vi "SplashWindow.vi"(7 "Name (\"\" to Use UUID)":string="SplashWindow") -> ()   [LabVIEW 2020, in "CSM-SplashWindow.lvlib"]
doc: "------------- lvcsm -------------\n[CSMStates]\nItem 0 = \"Idle\"\nItem 1 = \"CSM Documentation\"\nItem 2 = \"VI Reference\"\nItem 3 = \"Error Handler\"\nItem 4 = \"Critical Error\"\nItem 5 = \"Target Timeout Error\"\nItem 6 = \"Target Error\"\nItem 7 = \"Async Response\"\nItem 8 = \"Response\"\nItem 9 = \"Async Message Posted\"\nItem 10 = \"Initialize Core Data\"\nItem 11 = \"Exit\"\nItem 12 = \"Data: Initialize\"\nItem 13 = \"Data: Update Indicators\"\nItem 14 = \"Data: Cleanup\"\nItem 15 = \"Macro: Initialize\"\nItem 16 = \"Macro: Exit\"\nItem 17 = \"API: Information Handler\"\nItem 18 = \"API: Module Starting Up Handler\"\nItem 19 = \"API: Update Title\"\nItem 20 = \"API: SplashWnd for Module Starting Up\"\nItem 21 = \"Action: Splash Msg\"\n\n[CSMStatus]\nItem 0 = \"Error Occurred@Error Handler\""
uses:
  <userlib>/_NEVSTOP/Communicable State Machine(CSM)/_Support/Typedef/_CSM_List Module Scope.ctl
  aaaf7aa3-717b-40f6-b678-5a45a36f8c0a.vi
  34a7b652-a0e3-4533-9b0d-8286918f5116.vi
  <userlib>/_NEVSTOP/Communicable State Machine(CSM)/_Shared/Trim Single-line Text.vi
  <userlib>/_NEVSTOP/Communicable State Machine(CSM)/AdvanceAPI/CSM - Make String Arguments Safe.vi
  <userlib>/_NEVSTOP/Communicable State Machine(CSM)/AdvanceAPI/CSM - Break Down Multiple States String.vi
  <userlib>/_NEVSTOP/Communicable State Machine(CSM)/AdvanceAPI/CSM - Compact Multiple States.vi
  <userlib>/_NEVSTOP/Communicable State Machine(CSM)/AdvanceAPI/CSM - Keywords.vi
  <userlib>/_NEVSTOP/Communicable State Machine(CSM)/_Support/Common/Format Timestamp.vi
  <userlib>/_NEVSTOP/Communicable State Machine(CSM)/_Polymophic/Add State(s) to Queue By BOOL(Element).vi
  <userlib>/_NEVSTOP/Communicable State Machine(CSM)/addons/API-String-Arugments-Support/_Support/Convert API String Arguments to Data(variant).vi
  CSM-SplashWindow.lvlib
  <userlib>/_NEVSTOP/Communicable State Machine(CSM)/Communicable State Machine.lvlib
panel:
  out "Title":string
  out "Error Occurred":errorcluster
  out "Message":string
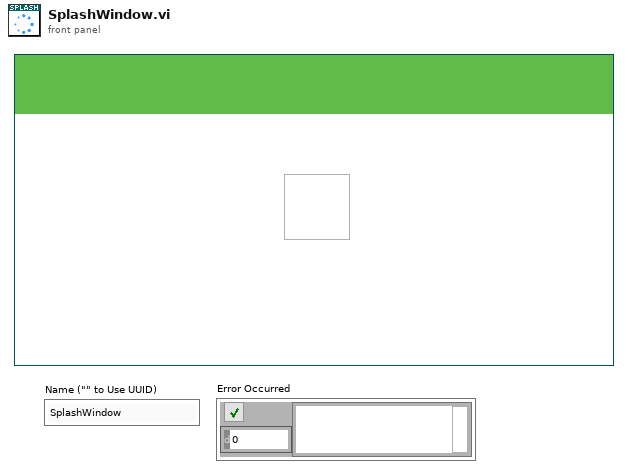
[diagram p1: front panel]
types:
  T1 = enum32{"Invalid", "Standard", "Closed", "Hidden", "Minimized", "Maximized"}
  T2 = enum32{"invalid app kind", "Development System", "Run Time System", "Student Edition", "Embedded LabVIEW", "Evaluation", "Custom"}
  T3 = typedef "Communicable State Machine.lvlib/_CSM_List Module Scope.ctl" = enum16{"Normal", "System Only", "All"}
  T4 = typedef "Communicable State Machine.lvlib/_CSM_Response Source Message.ctl" = cluster{"‘State":string, "’Arguments":string, "’Error":errorcluster}
  T5 = cluster{"Current VI Reference":refnum<vi>, "Close Panel on Exit?":bool}
  T6 = cluster{"Core":cluster{"Current VI Reference":refnum<vi>, "Close Panel on Exit?":bool}, "Your Boolean data":bool, "Modules":string[]}
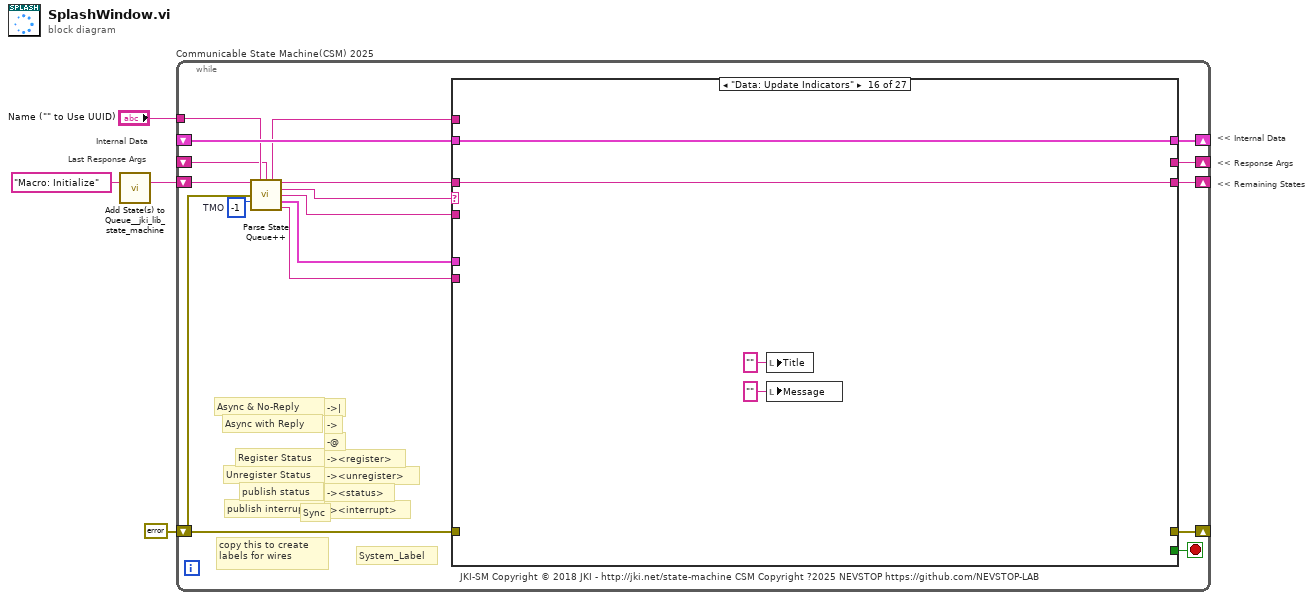
[diagram p0: block diagram]
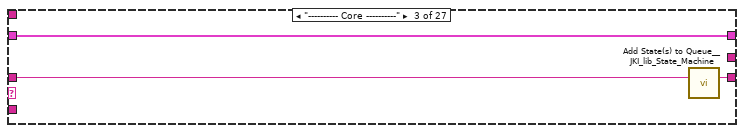
[diagram p4: hidden frame]
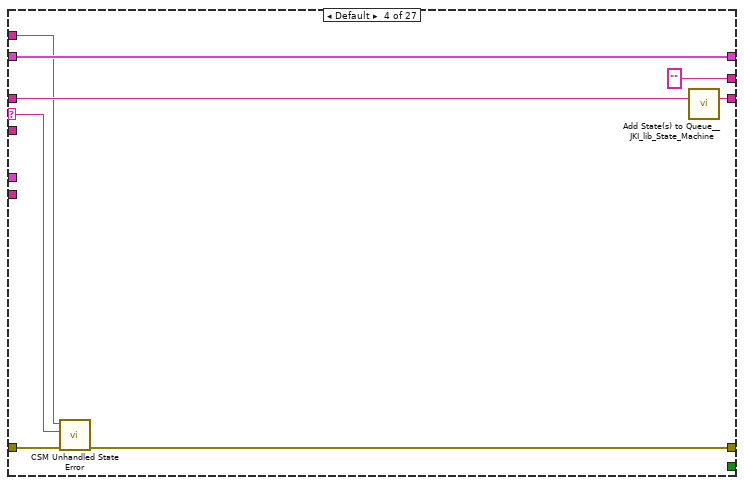
[diagram p5: hidden frame]
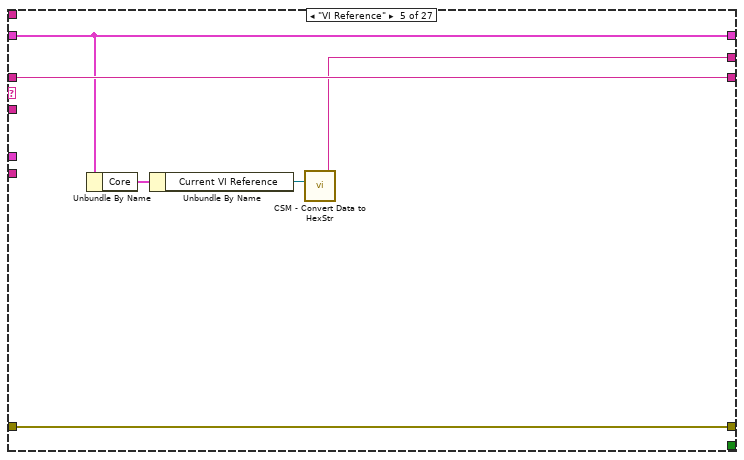
[diagram p6: hidden frame]
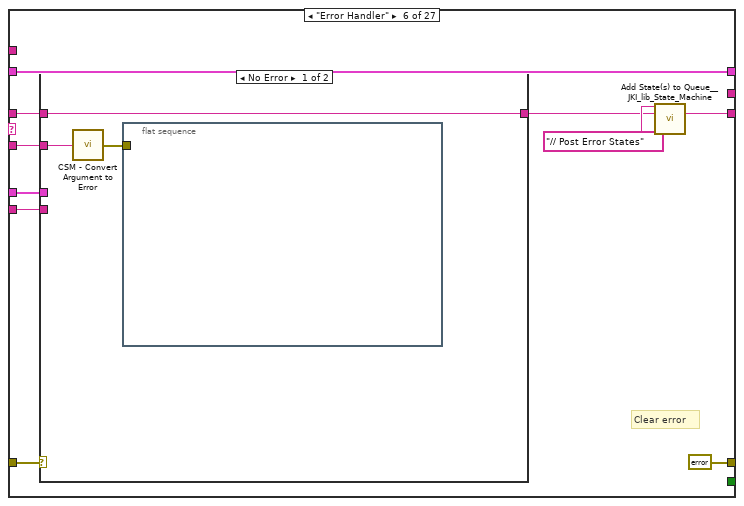
[diagram p7: hidden frame]
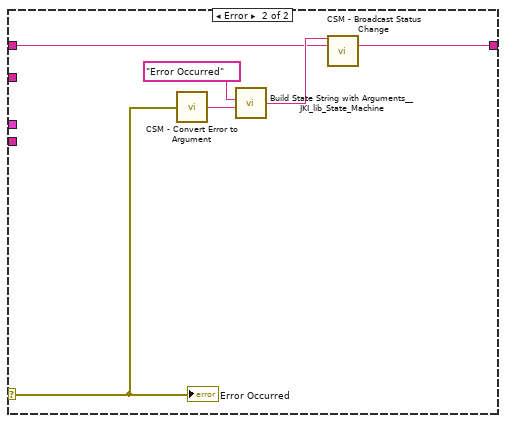
[diagram p8: hidden frame]
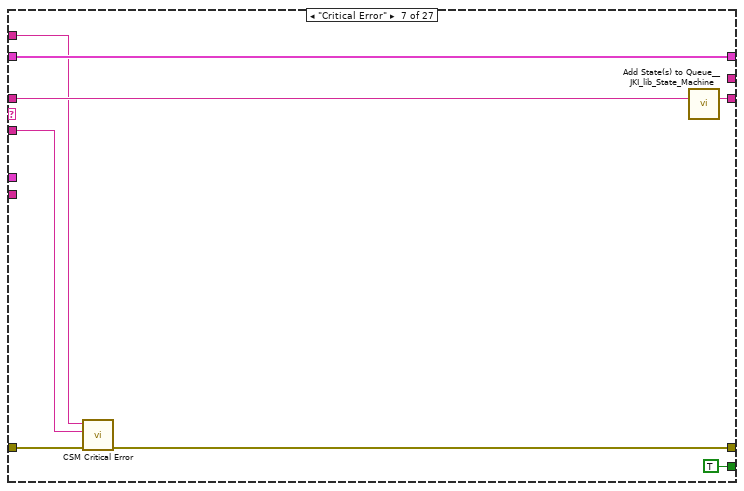
[diagram p9: hidden frame]
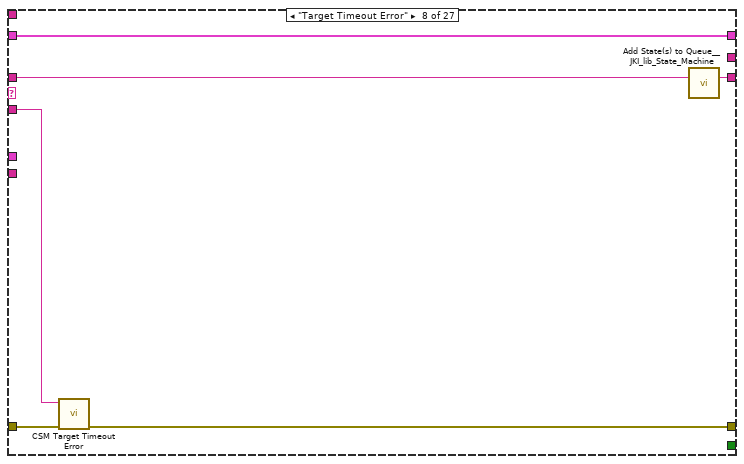
[diagram p10: hidden frame]
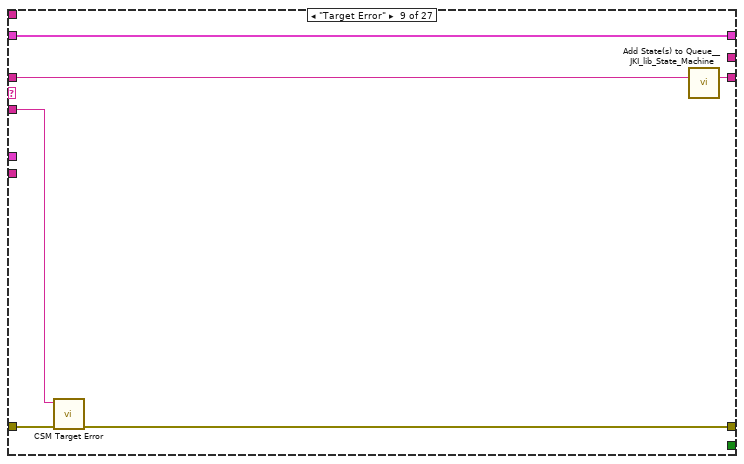
[diagram p11: hidden frame]
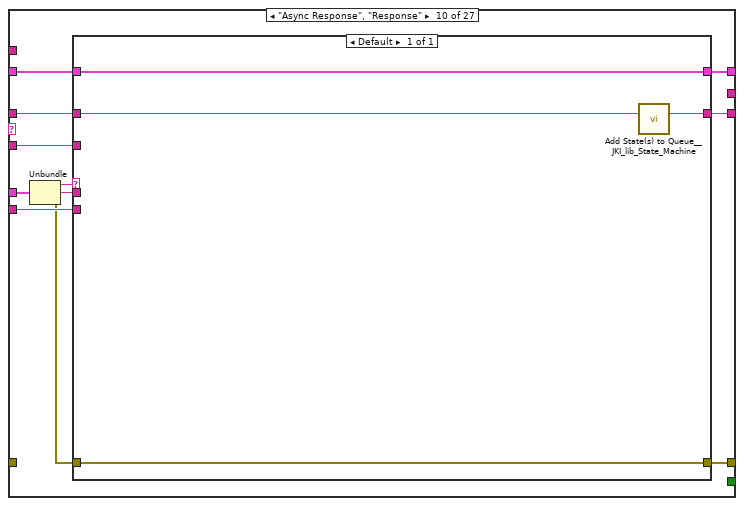
[diagram p12: hidden frame]
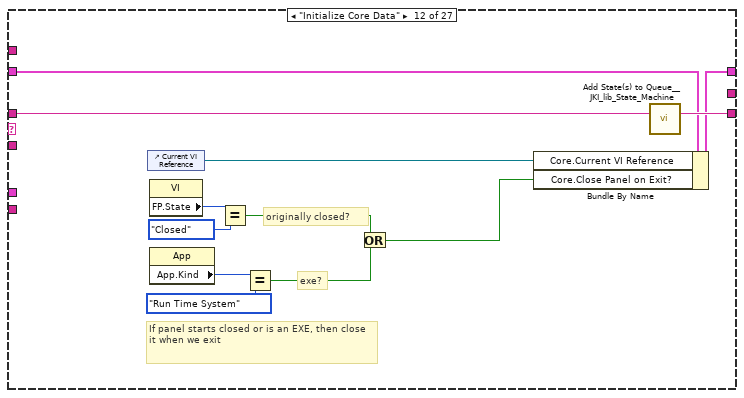
[diagram p14: hidden frame]
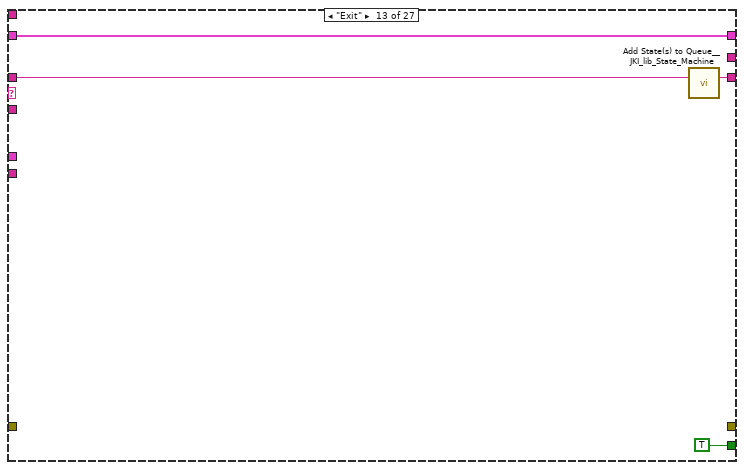
[diagram p15: hidden frame]
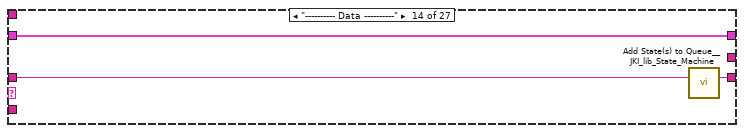
[diagram p16: hidden frame]
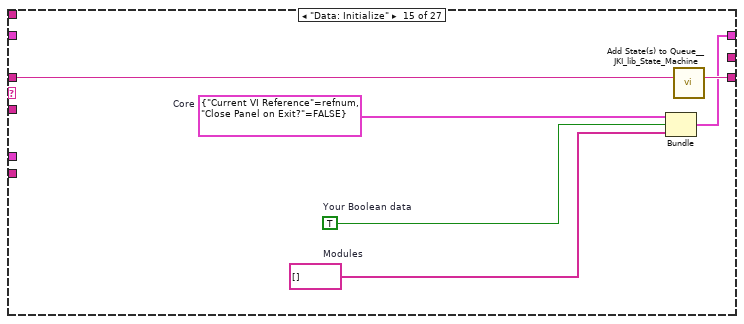
[diagram p17: hidden frame]
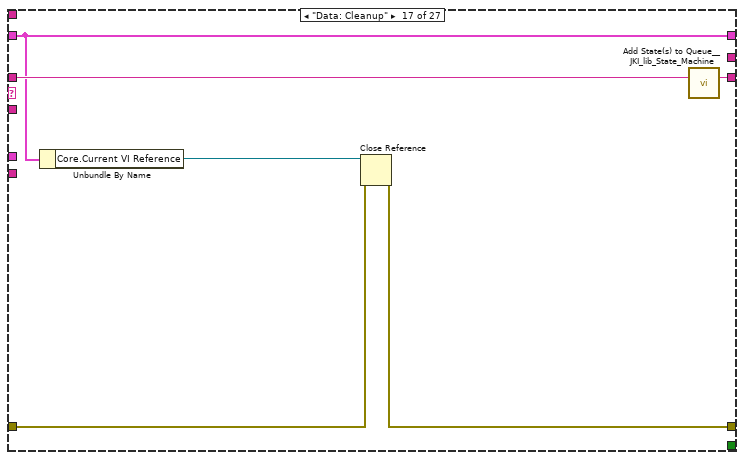
[diagram p18: hidden frame]
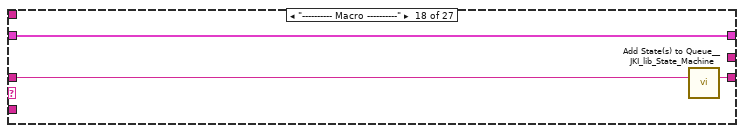
[diagram p19: hidden frame]
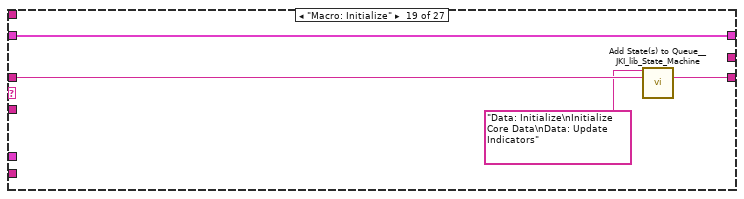
[diagram p20: hidden frame]
diagram:
  # "Last Response Args"
  # "Internal Data"
  # "<< Internal Data"
  # "<< Response Args"
  # "<< Remaining States"
  n1 = call <vilib>:"Add State(s) to Queue__jki_lib_state_machine.vi"("State(s) in (\"\")"="Macro: Initialize" ("Init State(\"Macro: Initialize\")")) -> ("States Out"=w2:string)  [unwired: 14 in]
  n2 = while "Communicable State Machine(CSM) 2025" {
    shift-right: [w16] -> _
    shift-left: _ -> [w15]
    shift-right: [w19] -> _
    shift-left: errorcluster {"status"=FALSE, "code"=0, "source"=""} ("error out") -> [w5]
    shift-right: [w18] -> _
    shift-left: w2 -> [w20]
    tunnel: "Name (\"\" to Use UUID)" -> [w12]
    shift-right: [w13] -> _
    shift-left: _ -> [w7]
    stop <- w17 stop-if-true
    w14 = -1  # TMO
    # "-><interrupt>"
    # "-><status>"
    # "-><unregister>"
    # "-><register>"
    # "-@"
    # "->"
    # "->|"
    # "publish interrupt"
    # "publish status"
    # "Unregister Status"
    # "Register Status"
    # "Sync"
    # "Async with Reply"
    # "Async & No-Reply"
    # "JKI-SM Copyright © 2018 JKI - http://jki.net/state-machine CSM Copyright ?2025 NEVSTOP https://github.com/NEVSTOP-LAB"
    # "copy this to create labels for wires"
    # "System_Label"
    n3 = call <userlib>:"Parse State Queue++.vi"("State Queue"=w20, "Name (\"\" to Use UUID)"=w12, "Response Arguments"=w7, "Previous Error"=w5, "Dequeue (1 ms)"=w14) -> ("Name Used"=w6:string, "Remaining States"=w21:string, "Current State"=w8:string, "Arguments"=w9:string, "Additional Information"=w10:T4, "Source CSM"=w11:string)  [unwired: 5 in]
    n4 = case shown="\"Data: Update Indicators\"" w8 {
      selector: w8 -> [_ _ _ w32 _ _ _ _ _ _ _ _ _ _ _ _ _ _ _ _ _ _ _ _ _ _ _]
      tunnel: w21 -> [w22 w25 w28 w36 w41 w46 w69 w75 w81 w91 w98 w110 w114 w117 w123 w127 w133 w136 w140 w146 w148 w152 w168 w182 w185 w195 w202]
      tunnel: w9 -> [_ _ _ _ _ w45 w65 w72 w78 w85 _ _ _ _ _ _ _ _ _ _ _ w149 _ w180 w190 _ w198]
      tunnel: w15 -> [w23 w24 w26 w34 w40 w51 w67 w73 w79 w89 w97 w104 w112 w115 _ w126 w128 w134 w138 w144 w147 w154 w165 w181 w191 w193 w200]
      tunnel: [_ _ _ w29 w42 errorcluster {"status"=FALSE, "code"=0, "source"=""} ("error out") w62 w70 w76 w92 _ _ _ _ _ _ w129 _ _ _ _ _ w174 w183 w192 _ _] -> w19
      tunnel: w5 -> [_ _ _ w30 w42 w49 w63 w71 w77 _ _ _ _ _ _ _ w130 _ _ _ _ _ w174 w183 w192 _ _]
      tunnel: [w22 w25 w27 w35 w41 w47 w68 w74 w80 w90 w98 w109 w113 w116 w122 w127 w132 w135 w139 w145 w148 w153 w157 w182 w186 w194 w201] -> w18
      tunnel: [_ _ _ _ _ _ TRUE _ _ _ _ _ TRUE _ _ _ _ _ _ _ _ _ _ _ _ _ _] -> w17
      tunnel: [w23 w24 w26 w34 w40 w51 w67 w73 w79 w88 w97 w108 w112 w115 w121 w126 w128 w134 w138 w144 w147 w154 w165 w181 w188 w193 w200] -> w16
      tunnel: w11 -> [_ _ _ _ _ w44 _ _ _ w86 _ _ _ _ _ _ _ _ _ _ _ _ w171 _ _ _ _]
      tunnel: w10 -> [_ _ _ _ _ w43 _ _ _ w87 _ _ _ _ _ _ _ _ _ _ _ _ _ _ _ _ _]
      tunnel: [_ _ _ "" w37 _ _ _ _ _ _ _ _ _ _ _ _ _ _ _ _ _ _ _ _ _ _] -> w13
      tunnel: w6 -> [_ _ _ w31 _ _ w64 _ _ _ _ _ _ _ _ _ _ _ _ _ _ _ _ _ _ _ _]
      frame "", "Idle" {
      }
      frame "CSM Documentation" {
      }
      frame "---------- Core ----------" {
        n5 = call <vilib>:"Add State(s) to Queue__JKI_lib_State_Machine.vi"("State(s) in (\"\")"=w28) -> ("States Out"=w27:string)  [unwired: 14 in]
      }
      frame Default {
        n6 = call <userlib>:"CSM Unhandled State Error.vi"("error in (no error)"=w30, "Undefined State"=w32, "CSM Name"=w31) -> ("error out"=w29:errorcluster)  [unwired: 8 in]
        n7 = call <vilib>:"Add State(s) to Queue__JKI_lib_State_Machine.vi"("State(s) in (\"\")"=w36) -> ("States Out"=w35:string)  [unwired: 14 in]
      }
      frame "VI Reference" {
        n8 = Unbundle By Name(w40) -> ("Core"=w39:T5)
        n9 = Unbundle By Name(w39) -> ("Current VI Reference"=w38:refnum<vi>)
        n10 = call <userlib>:"CSM - Convert Data to HexStr.vi"("Variant"=w38) -> ("HEX String (0-9,A-F)"=w37:string)  [unwired: 8 in]
      }
      frame "Error Handler" {
        # "Clear error"
        n11 = case shown="No Error" w49 {
          selector: w49 -> [_ w56]
          tunnel: [w55 w58] -> w48
          tunnel: w46 -> [w55 w57]
          tunnel: w45 -> [w54 _]
          tunnel: w44 -> [_ _]
          tunnel: w43 -> [_ _]
          frame No Error {
            n12 = call <userlib>:"CSM - Convert Argument to Error.vi"("Argument"=w54) -> ("Error"=w53:errorcluster)  [unwired: 4 in]
            n13 = flat-sequence {
              tunnel: w53 -> [_]
              frame #0 {
              }
            }
          }
          frame Error {
            n14 = call <userlib>:"CSM - Convert Error to Argument.vi"("Error"=w56) -> ("Argument"=w60:string)  [unwired: 4 in]
            n15 = call <vilib>:"Build State String with Arguments__JKI_lib_State_Machine.vi"("Arguments (\"\")"=w60, "State"="Error Occurred" ("Status with Arguments")) -> ("State with Arguments"=w59:string)  [unwired: 4 in]
            n16 = call <userlib>:"CSM - Broadcast Status Change.vi"("Status With Arguments"=w59, "State Queue"=w57) -> ("Remaining States"=w58:string)  [unwired: 13 in]
            "Error Occurred" <- w56
          }
        }
        n17 = call <vilib>:"Add State(s) to Queue__JKI_lib_State_Machine.vi"("State(s) in Front (\"\")"="// Post Error States", "State(s) in (\"\")"=w48) -> ("States Out"=w47:string)  [unwired: 13 in]
      }
      frame "Critical Error" {
        n18 = call <userlib>:"CSM Critical Error.vi"("error in (no error)"=w63, "Arugments (As Reason)"=w65, "CSM Name"=w64) -> ("error out"=w62:errorcluster)  [unwired: 8 in]
        n19 = call <vilib>:"Add State(s) to Queue__JKI_lib_State_Machine.vi"("State(s) in (\"\")"=w69) -> ("States Out"=w68:string)  [unwired: 14 in]
      }
      frame "Target Timeout Error" {
        n20 = call <userlib>:"CSM Target Timeout Error.vi"("error in (no error)"=w71, "Arguments (As CSM Name)"=w72) -> ("error out"=w70:errorcluster)  [unwired: 9 in]
        n21 = call <vilib>:"Add State(s) to Queue__JKI_lib_State_Machine.vi"("State(s) in (\"\")"=w75) -> ("States Out"=w74:string)  [unwired: 14 in]
      }
      frame "Target Error" {
        n22 = call <userlib>:"CSM Target Error.vi"("error in (no error)"=w77, "Arguments (As CSM Name)"=w78) -> ("error out"=w76:errorcluster)  [unwired: 9 in]
        n23 = call <vilib>:"Add State(s) to Queue__JKI_lib_State_Machine.vi"("State(s) in (\"\")"=w81) -> ("States Out"=w80:string)  [unwired: 14 in]
      }
      frame "Async Response", "Response" {
        n24 = Unbundle(w87) -> ("‘State"=w84:string, "’Arguments"=w83:string, "’Error"=w82:errorcluster)
        n25 = case shown="Default" w84 {
          tunnel: [w93] -> w90
          tunnel: w91 -> [w94]
          tunnel: [w96] -> w88
          tunnel: w89 -> [w96]
          tunnel: [w95] -> w92
          tunnel: w82 -> [w95]
          tunnel: w86 -> [_]
          tunnel: w85 -> [_]
          tunnel: w83 -> [_]
          frame Default {
            n26 = call <vilib>:"Add State(s) to Queue__JKI_lib_State_Machine.vi"("State(s) in (\"\")"=w94) -> ("States Out"=w93:string)  [unwired: 14 in]
          }
        }
      }
      frame "Async Message Posted" {
      }
      frame "Initialize Core Data" {
        # "originally closed?"
        # "exe?"
        # "If panel starts closed or is an EXE, then close it when we exit"
        n27 = control-ref of="Current VI Reference"() -> (w102:refnum<vi>)
        n28 = property class="VI"() -> ("FP.State"=w101:T1)  [unwired: 2 in, 2 out]
        n29 = property class="App"() -> ("App.Kind"=w107:T2)  [unwired: 2 in, 2 out]
        n30 = Equal?(x=w101, y=T1."Closed" ("Front Panel Window:State")) -> (x = y?=w99:bool)
        n31 = Equal?(x=w107, y=T2."Run Time System" ("Application:Kind")) -> (x = y?=w105:bool)
        n32 = Or(x=w99, y=w105) -> (x .or. y?=w103:bool)
        n33 = Bundle By Name(cluster=w104, "Core.Current VI Reference"=w102, "Core.Close Panel on Exit?"=w103) -> (w108:T6)
        n34 = call <vilib>:"Add State(s) to Queue__JKI_lib_State_Machine.vi"("State(s) in (\"\")"=w110) -> ("States Out"=w109:string)  [unwired: 14 in]
      }
      frame "Exit" {
        n35 = call <vilib>:"Add State(s) to Queue__JKI_lib_State_Machine.vi"("State(s) in (\"\")"=w114) -> ("States Out"=w113:string)  [unwired: 14 in]
      }
      frame "---------- Data ----------" {
        n36 = call <vilib>:"Add State(s) to Queue__JKI_lib_State_Machine.vi"("State(s) in (\"\")"=w117) -> ("States Out"=w116:string)  [unwired: 14 in]
      }
      frame "Data: Initialize" {
        w118 = T5 {"Current VI Reference"=refnum, "Close Panel on Exit?"=FALSE}  # Core
        w120 = TRUE  # Your Boolean data
        w119 = string[] []  # Modules
        n37 = Bundle("Core"=w118, "Your Boolean data"=w120, "Modules"=w119) -> (w121:T6)  [unwired: 1 in]
        n38 = call <vilib>:"Add State(s) to Queue__JKI_lib_State_Machine.vi"("State(s) in (\"\")"=w123) -> ("States Out"=w122:string)  [unwired: 14 in]
      }
      frame "Data: Update Indicators" {
        n39 = local write "Title"("" ("Title")) -> ()
        n40 = local write "Message"("" ("Title")) -> ()
      }
      frame "Data: Cleanup" {
        n41 = Unbundle By Name(w128) -> ("Core.Current VI Reference"=w131:refnum<vi>)
        n42 = Close Reference(reference=w131, error in (no error)=w130) -> (error out=w129:errorcluster)
        n43 = call <vilib>:"Add State(s) to Queue__JKI_lib_State_Machine.vi"("State(s) in (\"\")"=w133) -> ("States Out"=w132:string)  [unwired: 14 in]
      }
      frame "---------- Macro ----------" {
        n44 = call <vilib>:"Add State(s) to Queue__JKI_lib_State_Machine.vi"("State(s) in (\"\")"=w136) -> ("States Out"=w135:string)  [unwired: 14 in]
      }
      frame "Macro: Initialize" {
        n45 = call <vilib>:"Add State(s) to Queue__JKI_lib_State_Machine.vi"("State(s) in Front (\"\")"="Data: Initialize\nInitialize Core Data\nData: Update Indicators", "State(s) in (\"\")"=w140) -> ("States Out"=w139:string)  [unwired: 13 in]
      }
      frame "Macro: Exit" {
        n46 = call <vilib>:"Add State(s) to Queue__JKI_lib_State_Machine.vi"("State(s) in Front (\"\")"="//Exit Sub-Modules ", "State(s) at Back (\"\")"="Data: Cleanup\nExit") -> ("States Out"=w142:string)  [unwired: 13 in]
        n47 = call <vilib>:"Add State(s) to Queue__JKI_lib_State_Machine.vi"("State(s) in Front (\"\")"=w142, "State(s) in (\"\")"=w146) -> ("States Out"=w145:string)  [unwired: 13 in]
      }
      frame "---------- API ----------" {
      }
      frame "API: Information Handler" {
        n48 = call <vilib>:"Build State String with Arguments__jki_lib_state_machine.vi"("Arguments (\"\")"=w149, "State"="Action: Splash Msg" ("State(s) at Back (\"\")")) -> ("State with Arguments"=w150:string)  [unwired: 4 in]
        n49 = call <vilib>:"Add State(s) to Queue__jki_lib_state_machine.vi"("State(s) in (\"\")"=w152, "State(s) at Back (\"\")"=w150) -> ("States Out"=w153:string)  [unwired: 13 in]
      }
      frame "API: Module Starting Up Handler" {
        n50 = Unbundle By Name(w165) -> ("Modules"=w163:string[])
        n51 = call <userlib>:"CSM - List Modules.vi"("Scope (Normal)"=_CSM_List_Module_Scope."All") -> ("Module Names"=w164:string[])  [unwired: 9 in, 1 out]
        n52 = To Lower Case(string=w163) -> (all lower case string=w161:string[])
        n53 = To Lower Case(string=w164) -> (all lower case string=w162:string[])
        n54 = Format Into String(format string="\"%s\" is initialized..", w171) -> (resulting string=w170:string)  [unwired: 2 in, 1 out]
        n55 = for {
          tunnel: w162 -> [w178]
          tunnel: w161 -> [w177] mode=indexing
          tunnel: [w175] -> w160 mode=indexing
          n56 = Search 1D Array(1D array=w178, element=w177) -> (index of element=w176:i32)  [unwired: 1 in]
          n57 = Greater Or Equal To 0?(x=w176) -> (x >= 0?=w175:bool)
        }
        n58 = call <vilib>:"Build State String with Arguments__jki_lib_state_machine.vi"("Arguments (\"\")"=w170, "State"="Action: Splash Msg" ("State(s) at Back (\"\")")) -> ("State with Arguments"=w167:string)  [unwired: 4 in]
        n59 = And Array Elements(Boolean array=w160) -> (logical AND=w159:bool)
        n60 = call "Not Empty Array_nevstop.vim"("Array"=w160) -> ("not empty?"=w158:bool)
        n61 = And(x=w158, y=w159) -> (x .and. y?=w156:bool)
        n62 = call <vilib>:"Add State(s) to Queue__jki_lib_state_machine.vi"("State(s) in Front (\"\")"=w167, "State(s) in (\"\")"=w168) -> ("States Out"=w169:string)  [unwired: 13 in]
        n63 = call-poly <userlib>:"Add State(s) to Queue By BOOL++.vi"("TRUE (\"\")"="Macro: Exit" ("State(s) at Back (\"\")"), "Condition"=w156, "State Queue (\"\")"=w169) -> ("Remaining States"=w157:string)  [unwired: 8 in]
      }
      frame "API: Update Title" {
        n64 = call <userlib>:"CSM - Revert Arguments-Safe String.vi"("Safe Argument String"=w180) -> ("Origin Argument String"=→"Title":string)  [unwired: 8 in]
      }
      frame "API: SplashWnd for Module Starting Up" {
        n65 = call "Convert API String Arguments to Data.vim"("Reference Type"=string[] [] ("Init State(\"Macro: Initialize\")"), "API String"=w190) -> ("Data"=w187:string[])  [unwired: 6 in, 1 out]
        n66 = Bundle By Name(cluster=w191, "Modules"=w187) -> (w188:T6)
        n67 = call <vilib>:"Add State(s) to Queue__JKI_lib_State_Machine.vi"("State(s) in Front (\"\")"="Macro: Initialize@* >> API: Module Starting Up Handler -><register> " ("State(s) in Front (\"\")"), "State(s) in (\"\")"=w185) -> ("States Out"=w186:string)  [unwired: 13 in]
      }
      frame "---------- Action ----------" {
        n68 = call <vilib>:"Add State(s) to Queue__JKI_lib_State_Machine.vi"("State(s) in (\"\")"=w195) -> ("States Out"=w194:string)  [unwired: 14 in]
      }
      frame "Action: Splash Msg" {
        n69 = call <userlib>:"String History Cacher.vi"("Length"=1000 ("length (rest)"), "Include Timestamp? (T)"=FALSE, "String"=w198) -> ("String Cache"=→"Message":string)  [unwired: 8 in]
        n70 = call <vilib>:"Add State(s) to Queue__JKI_lib_State_Machine.vi"("State(s) in (\"\")"=w202) -> ("States Out"=w201:string)  [unwired: 14 in]
      }
    }
  }
